vi "data read.vi"() -> (3 "F-format string":string[](array[string]))   [LabVIEW 2019]
panel:
  out "status":dbl
  out "measurement data":dbl[](array[numeric]) format="%#_7p"
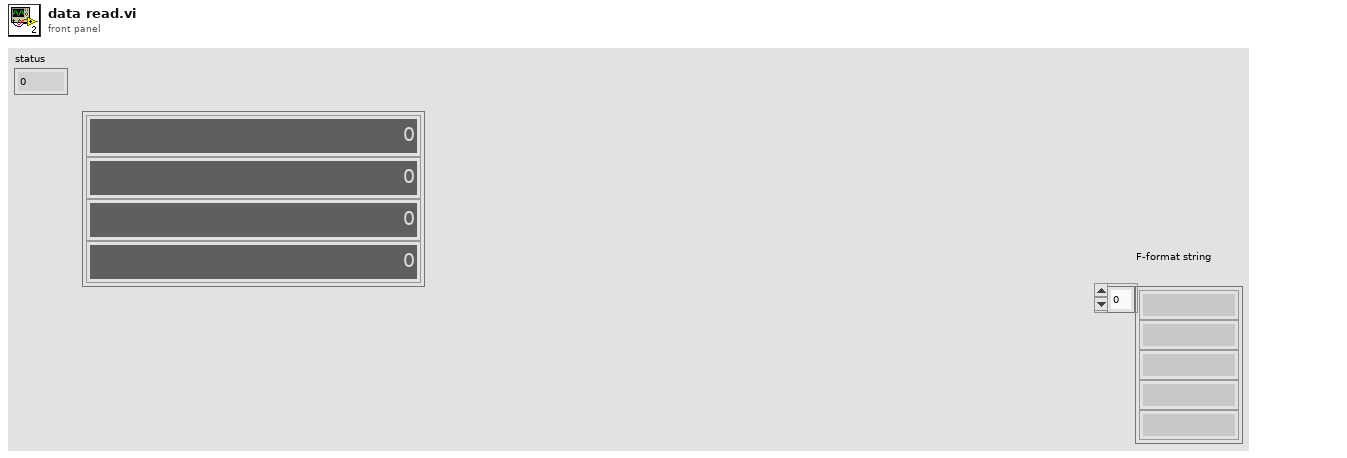
[diagram p1: front panel]
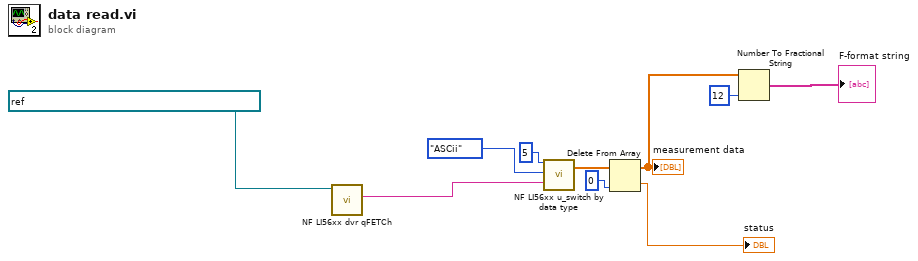
[diagram p0: block diagram]
diagram:
  n1 = call "NF LI56xx dvr qFETCh.vi"("VISA resource name"=refnum<visa-resource-name> "USB0::0x0D4A::0x004F::9253259::INSTR") -> ("measurement data"=w8:string)  [unwired: 8 in, 2 out]
  n2 = call "NF LI56xx u_switch by data type.vi"("Num"=u8 5 ("数値"), "data format"=enum16{"ASCii", "REAL", "INTeger"}."ASCii", "input string"=w8) -> ("query measurement data"=w7:dbl[])  [unwired: 16 in]
  n3 = Delete From Array(array=w7, index=0 ("指標")) -> (deleted portion=→"status":dbl, array with subset deleted=w4:dbl[])  [unwired: 1 in]
  "measurement data" <- w4
  n4 = Number To Fractional String(number=w4, precision (6)=i16 12) -> (F-format string=→"F-format string":string[])  [unwired: 2 in]
